vi "Get Statistics.vi"(8 "error in (no error)":errorcluster, 11 "Result Model in":refnum<class "Result Model by Reference.lvclass">) -> (0 "error out":errorcluster, 2 "Results":T1)   [LabVIEW 2020, in "Result Model by Reference.lvclass"]
uses:
  Result Model by Reference.lvclass
  Result Model/Statistics.ctl
  Result Model by Reference.lvclass/Result Model by Reference.ctl
  Result Model/Result Model.lvclass
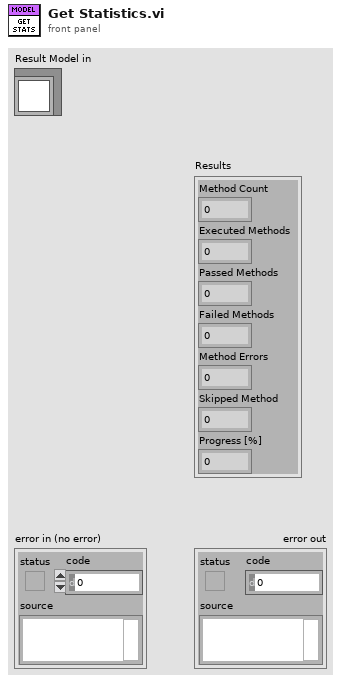
[diagram p1: front panel]
types:
  T1 = typedef "Result Model.lvclass/Statistics.ctl" = cluster{"Method Count":u32, "Executed Methods":u32, "Passed Methods":u32, "Failed Methods":u32, "Method Errors":u32, "Skipped Method":u32, "Progress [%]":dbl}
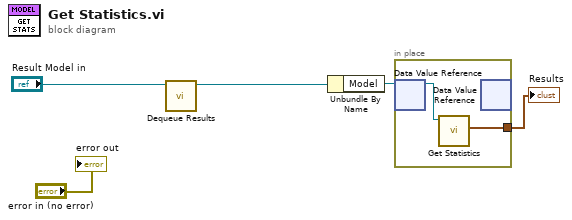
[diagram p0: block diagram]
diagram:
  n1 = call "Dequeue Results.vi"("Result Model by Reference in"="Result Model in") -> ("Result Model by Reference out"=w2:refnum<class "Result Model by Reference.lvclass">)  [unwired: 10 in]
  n2 = Unbundle By Name(w2) -> ("Model"=w5:refnum<data-value>)
  n3 = in-place {
    in-place-border: [w6] -> w3
    n4 = in-place-dvr #1(w5) -> (w7:refnum<class "Result Model.lvclass">)  [unwired: 1 out]
    n5 = call "Get Statistics.vi"("Result Model in"=w7) -> ("Results"=w6:T1)  [unwired: 10 in]
    n6 = in-place-dvr #1() -> ()  [unwired: 1 in, 2 out]
  }
  "Results" <- w3
  "error out" <- "error in (no error)"
